vi "Timer.vi"(1 "Wait Time (ms)":u32) -> (0 "Time Done":bool)   [LabVIEW 2012]
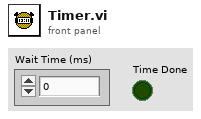
[diagram p1: front panel]
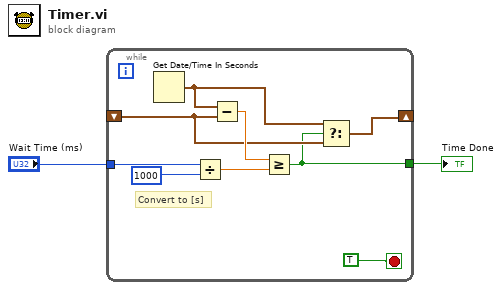
[diagram p0: block diagram]
diagram:
  n1 = while {
    shift-right: [w11] -> _
    shift-left: _ -> [w5]
    tunnel: "Wait Time (ms)" -> [w9]
    tunnel: [w4] -> w1
    stop <- TRUE stop-if-true
    # "Convert to [s]"
    n2 = Get Date/Time In Seconds() -> (seconds since 1Jan1904=w10:timestamp)
    n3 = Divide(x=w9, y=1000) -> (x/y=w6:dbl)
    n4 = Subtract(x=w10, y=w5) -> (x-y=w7:dbl)
    n5 = Greater Or Equal?(x=w7, y=w6) -> (x >= y?=w4:bool)
    n6 = Select(t=w10, s=w4, f=w5) -> (s? t:f=w11:timestamp)
  }
  "Time Done" <- w1
